vi "Save Archive Headers.vi"(8 "error in (no error)":errorcluster) -> (0 "error out":errorcluster)   [LabVIEW 2009]
uses:
  LogFileType.ctl
  NTCP Client/Control Point Suffix.ctl
  Data Access Objects/Metadata/Persistant DAO Actions.ctl
  Data Access Objects/Metadata/DAO Actions.ctl
panel:
  in  "LogFile Type":T1
  in  "Contol\nPoint\nSuffix":T2
  in  "Archive Headers":T1[](array[typedef])=[enum."Continuous", enum."Step", enum."Volts", enum."Offsets"]
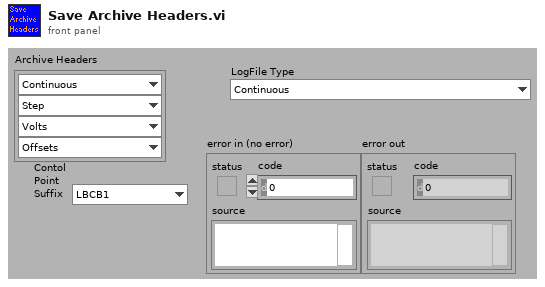
[diagram p1: front panel]
types:
  T1 = typedef "LogFileType.ctl" = enum16{"Continuous", "Step", "Volts", "Offsets", "Mixed Mode State", "DLL  Errors", "End List"}
  T2 = typedef "Control Point Suffix.ctl" = enum16{"LBCB1", "LBCB2", "ExternalSensors"}
  T3 = typedef "Persistant DAO Actions.ctl" = enum16{"Init", "Get", "Set", "Load", "Save"}
  T4 = typedef "App Parameters.ctl" = cluster{"Monitor Loop":T5, "Ramp Time":T5, "Log Loop":T5, "TCP to DAQ":T5, "Logging Directory":path, "Log File Size (MBytes)":i64, "Volt Logging Loop":T5}
  T5 = typedef "Timing Parameters.ctl" = cluster{"Interval":dbl, "Rate ":dbl}
  T6 = typedef "DAO Actions.ctl" = enum16{"Init", "Get", "Set"}
  T7 = enum16{"open", "replace", "create", "open or create", "replace or create", "replace or create with confirmation"}
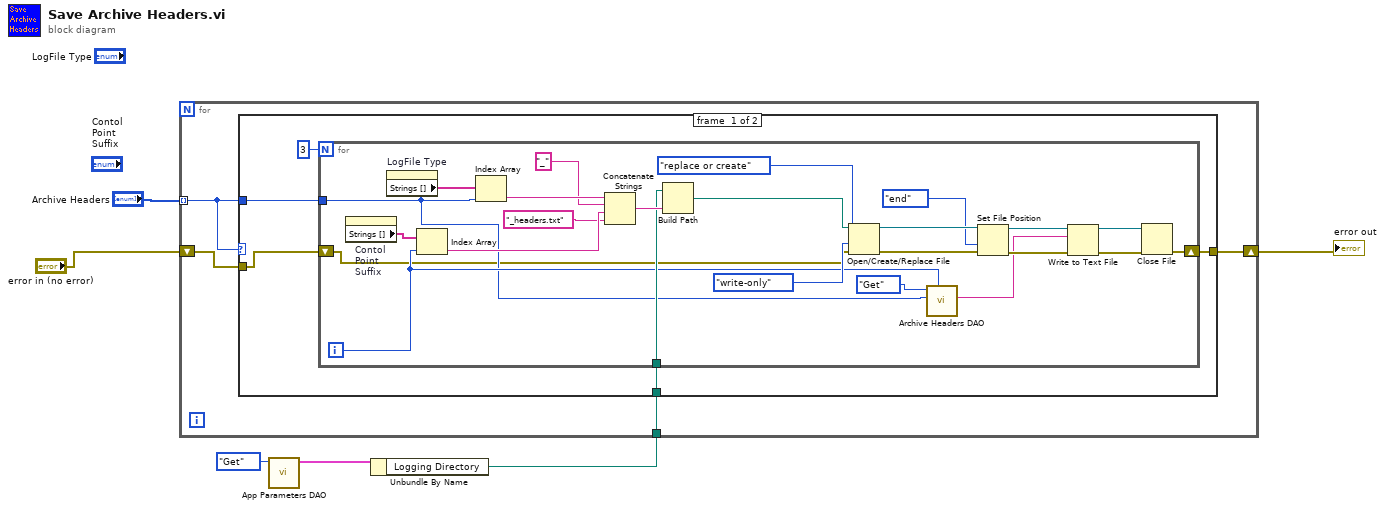
[diagram p0: block diagram]
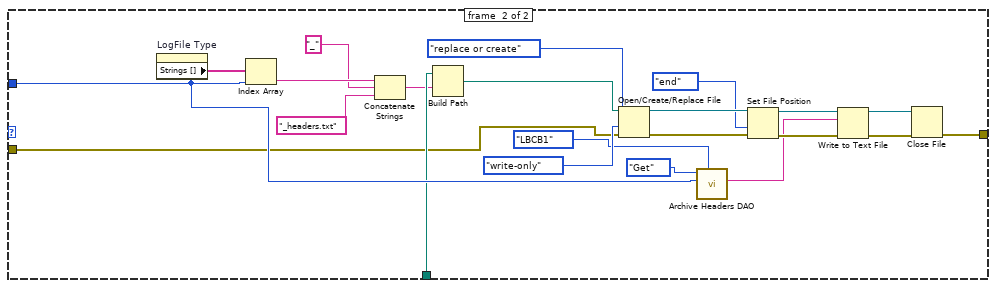
[diagram p2: hidden frame]
diagram:
  n1 = call "App Parameters DAO.vi"("Actions"=Persistant_DAO_Actions."Get") -> ("Application Timing and Logging Out"=w4:T4)  [unwired: 3 in, 7 out]
  n2 = Unbundle By Name(w4) -> ("Logging Directory"=w3:path)
  n3 = for {
    tunnel: "Archive Headers" -> [w9] mode=indexing
    tunnel: w3 -> [w10]
    shift-right: [w7] -> w1
    shift-left: "error in (no error)" -> [w8]
    n4 = case shown="\"Volts\"" w9 {
      tunnel: w9 -> [w14 w61]
      tunnel: w10 -> [w13 w60]
      tunnel: w8 -> [w12 w41]
      tunnel: [w11 w40] -> w7
      frame #0 {
        n5 = for {
          N: 3 -> [_]
          tunnel: w14 -> [w19]
          tunnel: w13 -> [w32]
          shift-right: [w16] -> w11
          shift-left: w12 -> [w17]
          i -> [w20]
          n6 = property on="Contol\nPoint\nSuffix" class="Enum (strict)"() -> ("Strings []"=w39:string[])  [unwired: 2 in, 2 out]
          n7 = property on="LogFile Type" class="Enum (strict)"() -> ("Strings []"=w38:string[])  [unwired: 2 in, 2 out]
          n8 = Index Array(array=w39, index=w20) -> (element=w35:string)
          n9 = Index Array(array=w38, index=w19) -> (element=w37:string)
          n10 = Concatenate Strings(w37, "_" ("string"), w35, "_headers.txt" ("string")) -> (w33:string)
          n11 = Build Path(base path=w32, name or relative path=w33) -> (appended path=w22:path)
          n12 = Open/Create/Replace File(file path (use dialog)=w22, error in=w17, operation (0:open)=T7."replace or create", access (0:read/write)=enum16{"read/write", "read-only", "write-only"}."write-only") -> (refnum out=w27:refnum<file>, error out=w26:errorcluster)  [unwired: 3 out]
          n13 = call "Archive Headers DAO.vi"("Contol\nPoint\nSuffix"=w20, "LogFile Type"=w19, "Actions"=DAO_Actions."Get") -> ("Record Out"=w18:string)  [unwired: 2 in, 6 out]
          n14 = Set File Position(refnum=w27, from (0:start)=enum16{"start", "end", "current"}."end", error in=w26) -> (refnum out=w24:refnum<file>, error out=w25:errorcluster)  [unwired: 1 out]
          n15 = Write to Text File(file (use dialog)=w24, text=w18, error in=w25) -> (refnum out=w29:refnum<file>, error out=w30:errorcluster)  [unwired: 2 out]
          n16 = Close File(refnum=w29, error in=w30) -> (error out=w16:errorcluster)  [unwired: 1 out]
        }
      }
      frame #1 {
        n17 = property on="LogFile Type" class="Enum (strict)"() -> ("Strings []"=w59:string[])  [unwired: 2 in, 2 out]
        n18 = Index Array(array=w59, index=w61) -> (element=w58:string)
        n19 = Concatenate Strings(w58, "_" ("string"), "_headers.txt" ("string")) -> (w55:string)
        n20 = Build Path(base path=w60, name or relative path=w55) -> (appended path=w45:path)
        n21 = Open/Create/Replace File(file path (use dialog)=w45, error in=w41, operation (0:open)=T7."replace or create", access (0:read/write)=enum16{"read/write", "read-only", "write-only"}."write-only") -> (refnum out=w50:refnum<file>, error out=w49:errorcluster)  [unwired: 3 out]
        n22 = call "Archive Headers DAO.vi"("Contol\nPoint\nSuffix"=Control_Point_Suffix."LBCB1" ("Contol\nPoint\nSuffix"), "LogFile Type"=w61, "Actions"=DAO_Actions."Get") -> ("Record Out"=w43:string)  [unwired: 2 in, 6 out]
        n23 = Set File Position(refnum=w50, from (0:start)=enum16{"start", "end", "current"}."end", error in=w49) -> (refnum out=w47:refnum<file>, error out=w48:errorcluster)  [unwired: 1 out]
        n24 = Write to Text File(file (use dialog)=w47, text=w43, error in=w48) -> (refnum out=w52:refnum<file>, error out=w53:errorcluster)  [unwired: 2 out]
        n25 = Close File(refnum=w52, error in=w53) -> (error out=w40:errorcluster)  [unwired: 1 out]
      }
    }
  }
  "error out" <- w1
